vi "Optical Flow Implementation(SubVI).vi"(5 "Image Out in":T1, 6 "Threshold":dbl(slide)=1.0 scale=0.0..20.0, 7 "Velocity Component 2 Out in":T1, 8 "error in (no error)":errorcluster, 9 "ROI Descriptor":T2 {"Contours"."Type" items=["No Selection", "Point", "Line", "Rectangle", "Oval", "Polygon", "Freehand Region", "Annulus", "Unused2", "Unused3", "Broken Line", "Freehand Line", "Rotated Rectangle"]}, 10 "Image Dst Out":T1, 11 "Refnum in":T1) -> (0 "error out":errorcluster, 1 "Velocity Component 2 Out out":T1, 2 "Image Out out":T1, 3 "Velocity Component 1 Out out":T1, 4 "Image":T1(plugin-control))   [LabVIEW 2014]
uses:
  <vilib>/vision/Image Controls.llb/IMAQ Image.ctl
  <vilib>/vision/NI_Vision_Development_Module.lvlib
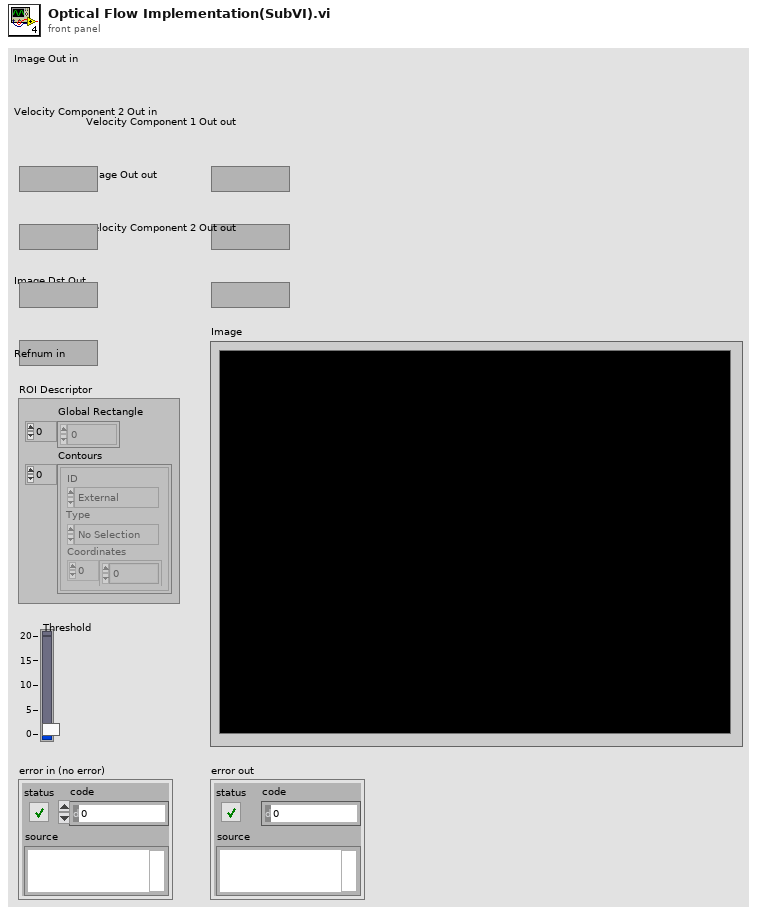
[diagram p1: front panel]
types:
  T1 = typedef "IMAQ Image.ctl" = refnum<image>
  T2 = typedef "ROI Descriptor" = cluster{"Global Rectangle":i32[], "Contours":cluster{"ID":enum32{"External", "Internal"}, "Type":u32, "Coordinates":i32[]}[]}
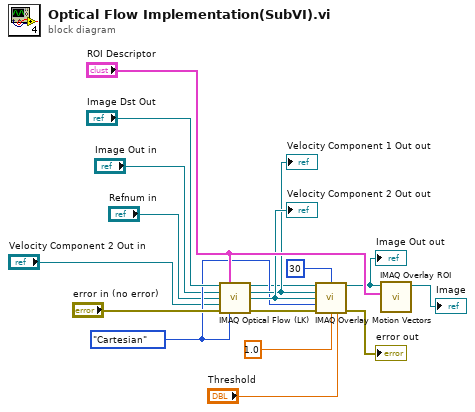
[diagram p0: block diagram]
diagram:
  w10 = enum16{"Cartesian", "Polar"}."Cartesian" ("Velocity Representation")
  n1 = call "IMAQ Optical Flow (LK)"("Current Frame"="Image Dst Out", "ROI Descriptor"="ROI Descriptor", "Previous Frame"="Image Out in", "Velocity Component 1 In"="Refnum in", "Velocity Component 2 In"="Velocity Component 2 Out in", "error in (no error)"="error in (no error)", "Velocity Representation"=w10) -> ("Current Frame Out (dup)"=w5:T1, "Velocity Component 1 Out"=w11:T1, "Velocity Component 2 Out"=w12:T1, "error out"=w4:errorcluster)  [unwired: 1 in, 4 out]
  "Velocity Component 2 Out out" <- w12
  "Velocity Component 1 Out out" <- w11
  n2 = call "IMAQ Overlay Motion Vectors"("Image"=w5, "Step Size"=30, "Velocity Component 1"=w11, "Velocity Component 2"=w12, "Velocity Representation"=w10, "error in (no error)"=w4, "Scale"=1.0, "Threshold"="Threshold") -> ("Image Out"=w15:T1, "error out"=→"error out":errorcluster)  [unwired: 2 in, 4 out]
  "Image Out out" <- w15
  n3 = call "IMAQ Overlay ROI"("ROI Descriptor"="ROI Descriptor", "Image"=w15) -> ("Image Out"=→"Image":T1)  [unwired: 8 in, 1 out]
